vi "PWM (SubVI).vi"(10 "Ciclo de Trabajo":dbl(knob) scale=0.0..100.0, 11 "Frecuencia":dbl(knob) scale=0.0..100.0) -> (3 "Señal PWM":dbl(graph))   [LabVIEW 2018]
doc: "Este VI funciona para escribir una señal PWM, con una frecuencia y ciclo de trabajo determinado por el usuario, en una grafica de tipo chart se muestra esta señal. Adicionalmente se añade un control para esperarse un número determinado de milisegundos y poder observar la señal.\n\nNota: Este VI debe introducirse en un ciclo while para escribir la señal de manera continúa.\n\n03-09-2024 \nRoberto Gómez Cruz"
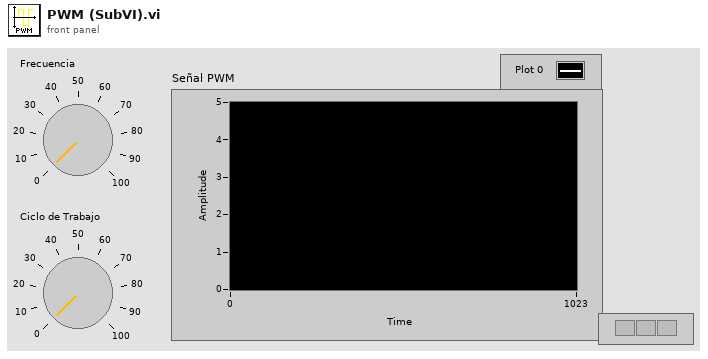
[diagram p1: front panel]
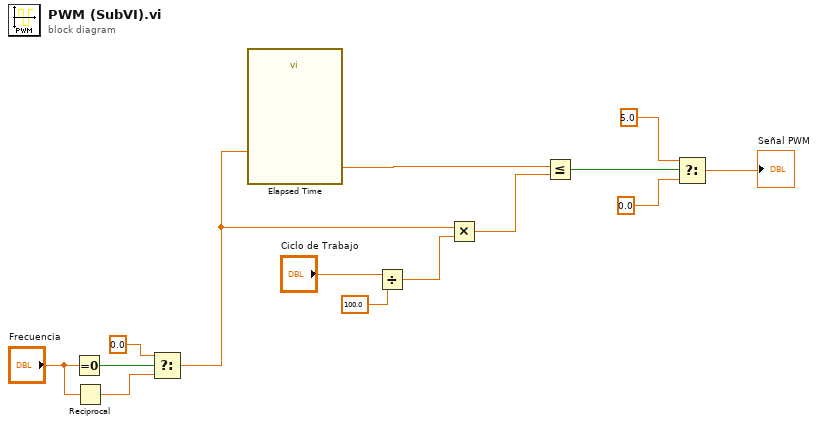
[diagram p0: block diagram]
diagram:
  n1 = Equal To 0?(x="Frecuencia") -> (x = 0?=w5:bool)
  n2 = Reciprocal(x="Frecuencia") -> (1/x=w2:dbl)
  n3 = Select(t=0.0, s=w5, f=w2) -> (s? t:f=w4:dbl)
  n4 = call "Elapsed Time"("Time Target (s)"=w4) -> ("Elapsed Time (s)"=w6:dbl)  [unwired: 11 in, 7 out]
  n5 = Divide(x="Ciclo de Trabajo", y=100.0) -> (x/y=w13:dbl)
  n6 = Multiply(x=w4, y=w13) -> (x*y=w7:dbl)
  n7 = Less Or Equal?(x=w6, y=w7) -> (x <= y?=w8:bool)
  n8 = Select(t=5.0, s=w8, f=0.0) -> (s? t:f=→"Señal PWM":dbl)
